vi "err dialog.vi"(10 "错误提示 2":errorcluster, 11 "参数 2":i32[](array[numeric])) -> ()   [LabVIEW 2009]
panel:
  in  "Boolean":bool
  out "参数":i32[](array[numeric])
  out "错误提示":errorcluster
  # "参数信息"
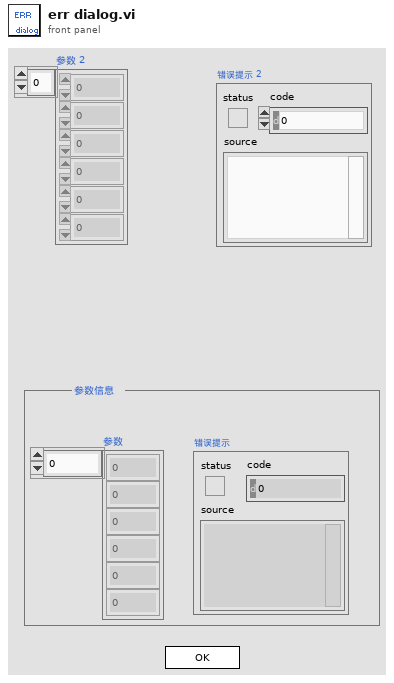
[diagram p1: front panel]
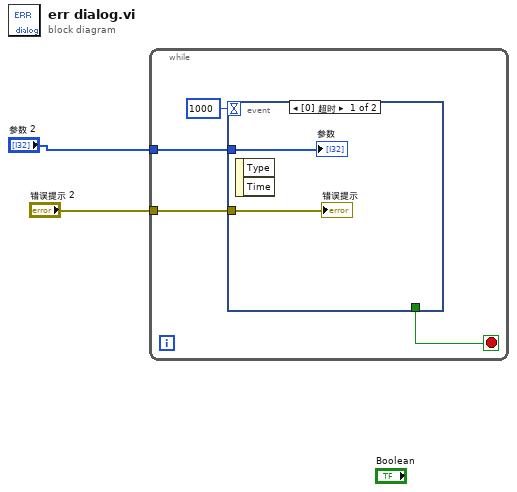
[diagram p0: block diagram]
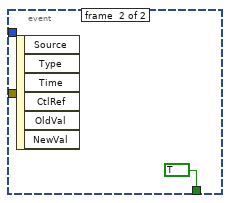
[diagram p2: hidden frame]
diagram:
  n1 = while {
    tunnel: "参数 2" -> [w6]
    tunnel: "错误提示 2" -> [w5]
    stop <- w4 stop-if-true
    n2 = event shown="[0] 超时" {
      selector: _ -> [_ _]
      dyn-events: _ -> [_ _]
      timeout: 1000 -> [_ _]
      tunnel: w6 -> [w8 _]
      tunnel: w5 -> [w7 _]
      tunnel: [_ TRUE] -> w4
      event #0 {
        n3 = event-data() -> ()  [unwired: 3 out]
        "参数" <- w8
        "错误提示" <- w7
      }
      event #1 {
        n4 = event-data() -> ()  [unwired: 7 out]
      }
    }
  }
